vi "03 - Demonstration - Dynamically Rebind Event Handlers.vi"() -> ()   [LabVIEW 2012]
panel:
  in  "Iterations":i32(ring)=20 items=["20"=20, "50"=50, "100"=100, "200"=200, "500"=500]
  in  "Rebind each iteration?":T1(ring)
  out "Subscriber B":i32(graph)
  out "Subscriber A":i32(graph)
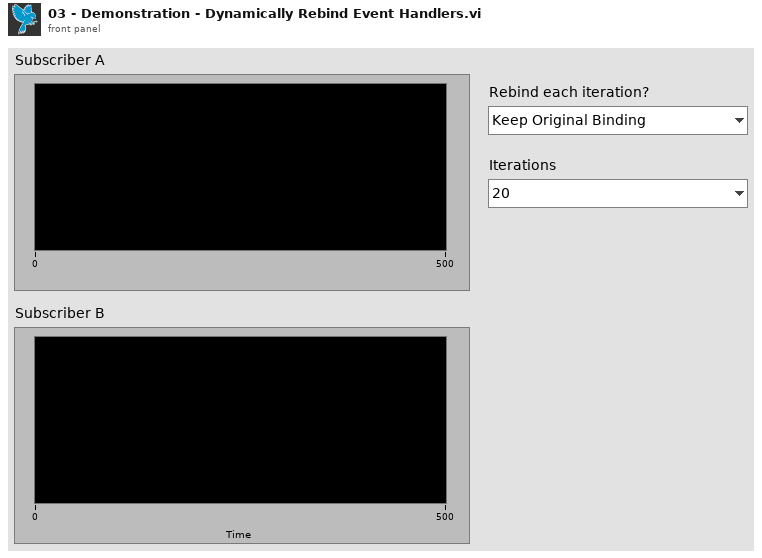
[diagram p1: front panel]
types:
  T1 = enum16{"Keep Original Binding", "Swap/Rebind Each Iteration"}
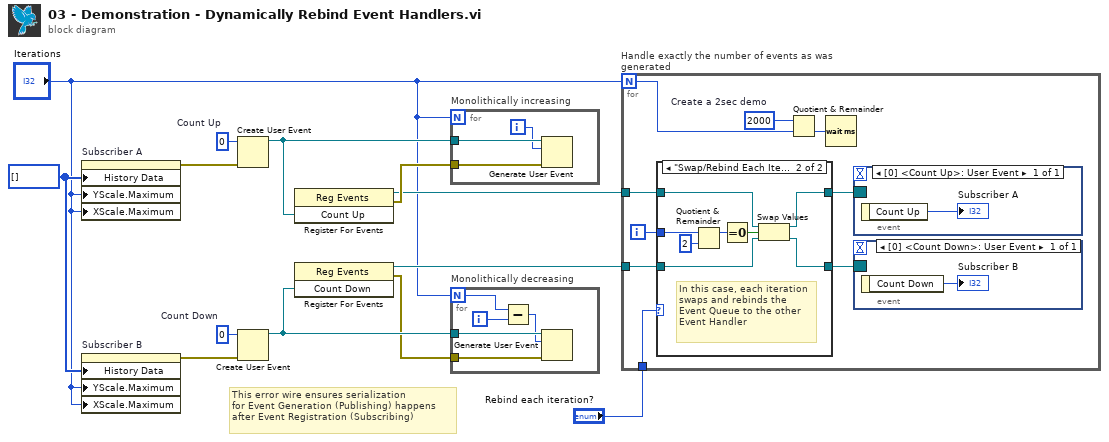
[diagram p0: block diagram]
diagram:
  w2 = i32[] [] ("History Data")
  w10 = 0  # Count Down
  w13 = 0  # Count Up
  # "This error wire ensures serialization\nfor Event Generation (Publishing) happens\nafter Event Registration (Subscribing)"
  n1 = property on="Subscriber A" class="WFChart (strict)"("History Data"=w2, "YScale.Maximum"="Iterations", "XScale.Maximum"="Iterations") -> (error out=w5:errorcluster)  [unwired: 2 in, 1 out]
  n2 = property on="Subscriber B" class="WFChart (strict)"("History Data"=w2, "YScale.Maximum"="Iterations", "XScale.Maximum"="Iterations") -> (error out=w3:errorcluster)  [unwired: 2 in, 1 out]
  n3 = Create User Event(user event datatype=w13, error in=w5) -> (user event=w11:refnum<user-event>)  [unwired: 1 out]
  n4 = Create User Event(user event datatype=w10, error in=w3) -> (user event=w9:refnum<user-event>)  [unwired: 1 out]
  n5 = register-events(w11) -> (reference out=w6:refnum<event-registration>, error out=w12:errorcluster)  [unwired: 2 in]
  n6 = register-events(w9) -> (reference out=w7:refnum<event-registration>, error out=w8:errorcluster)  [unwired: 2 in]
  n7 = for "Monolithically increasing" {
    N: "Iterations" -> [_]
    tunnel: w12 -> [w16]
    tunnel: w11 -> [w15]
    i -> [w14]
    n8 = Generate User Event(user event=w15, event data cluster=w14, error in=w16) -> ()  [unwired: 2 out]
  }
  n9 = for "Monolithically decreasing" {
    N: "Iterations" -> [w19]
    tunnel: w8 -> [w21]
    tunnel: w9 -> [w20]
    i -> [w17]
    n10 = Subtract(x=w19, y=w17) -> (x-y=w18:i32)
    n11 = Generate User Event(user event=w20, event data cluster=w18, error in=w21) -> ()  [unwired: 2 out]
  }
  n12 = for "Handle exactly the number of events as was generated" {
    N: "Iterations" -> [w24]
    tunnel: w7 -> [w28]
    tunnel: w6 -> [w29]
    tunnel: "Rebind each iteration?" -> [w25]
    i -> [w26]
    w23 = 2000  # Create a 2sec demo
    n13 = case shown="\"Swap/Rebind Each Iteration\"" w25 {
      tunnel: [w32 w39] -> w30
      tunnel: w29 -> [w32 w38]
      tunnel: w28 -> [w31 w37]
      tunnel: [w31 w36] -> w27
      tunnel: w26 -> [_ w34]
      frame "Keep Original Binding" {
      }
      frame "Swap/Rebind Each Iteration" {
        # "In this case, each iteration\nswaps and rebinds the\nEvent Queue to the other\nEvent Handler"
        n14 = Quotient & Remainder(x=w34, y=2) -> (x-y*floor(x/y)=w33:i32)  [unwired: 1 out]
        n15 = Equal To 0?(x=w33) -> (x = 0?=w35:bool)
        n16 = Swap Values(12:w38, 13:w35, 14:w37) -> (1:w39:refnum<event-registration>, 3:w36:refnum<event-registration>)
      }
    }
    n17 = Quotient & Remainder(x=w23, y=w24) -> (floor(x/y)=w22:i32)  [unwired: 1 out]
    n18 = Wait (ms)(milliseconds to wait=w22) -> ()  [unwired: 1 out]
    n19 = event shown="[0] <Count Up>: User Event" {
      selector: w30 -> [_]
      dyn-events: _ -> [_]
      timeout: _ -> [_]
      event User Event {
        n20 = event-data() -> ("Count Up"=→"Subscriber A":i32)  [unwired: 1 in]
      }
    }
    n21 = event shown="[0] <Count Down>: User Event" {
      selector: w27 -> [_]
      dyn-events: _ -> [_]
      timeout: _ -> [_]
      event User Event {
        n22 = event-data() -> ("Count Down"=→"Subscriber B":i32)  [unwired: 1 in]
      }
    }
  }
